vi "conector2.vi"(0 "salida":string[](array[string]), 1 "Salida ent":string, 2 "corriente entrada":dbl, 3 "polarizador":dbl[](array[numeric]), 4 "Polarizadorent":dbl, 5 "voltaje":dbl[](array[numeric]), 7 "VoltajeEnt":dbl, 8 "corrientes":dbl[](array[numeric]), 10 "Enum":T1(ring), 11 "Indice":i32) -> (12 "corrientes salida":dbl[](array[numeric]), 13 "VoltajeEnt 2":dbl, 14 "salida 2":string[](array[string]), 15 "Salida ent 2":string, 16 "corriente salida":dbl, 17 "polarizador 2":dbl[](array[numeric]), 18 "Polarizador":dbl, 19 "voltaje 2":dbl[](array[numeric]))   [LabVIEW 2016]
doc: "Este subVI selecciona al arreglo del cual se obtienen los valores que se enviarán a los dispositivos. \nLas entradas son tres arreglos y tres valores y de igual forma son las salidas."
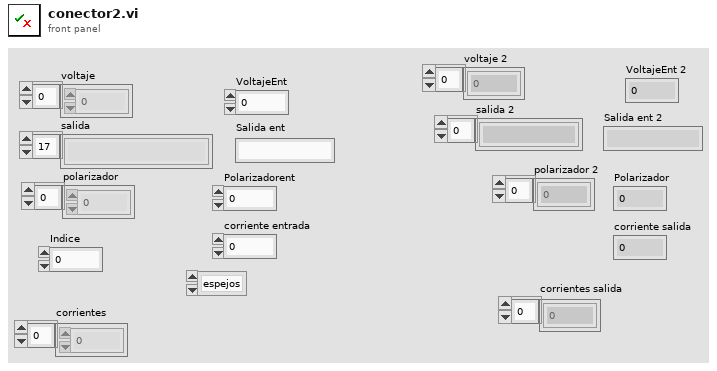
[diagram p1: front panel]
types:
  T1 = enum16{"espejos", "polarizador", "voltaje", "potenciometro ", "CCD", "lockin", "laser", "ninguno"}
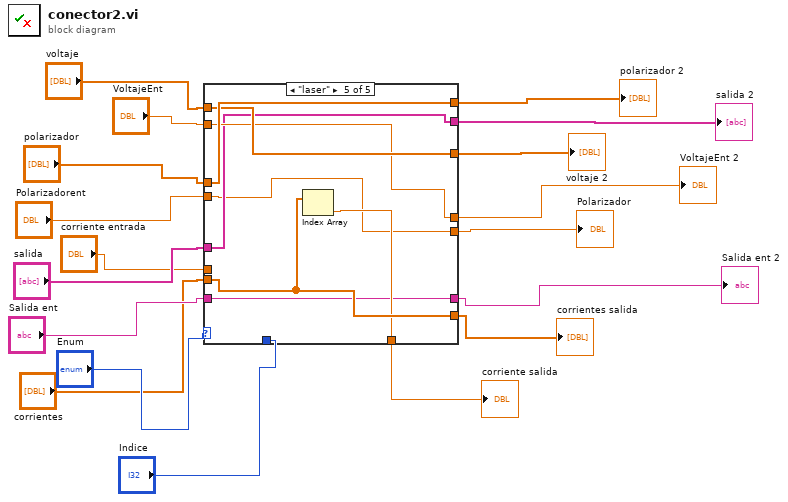
[diagram p0: block diagram]
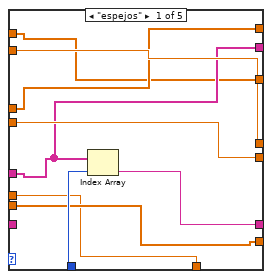
[diagram p2: hidden frame]
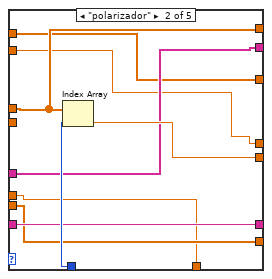
[diagram p3: hidden frame]
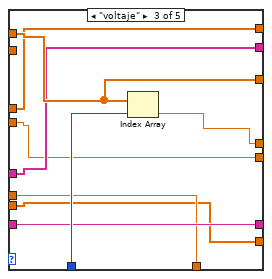
[diagram p4: hidden frame]
diagram:
  n1 = case shown="\"laser\"" "Enum" {
    tunnel: "polarizador" -> [w26 w34 w39 w53 w59]
    tunnel: "Indice" -> [w21 w36 w45 _ _]
    tunnel: [w25 w35 w40 w49 w55] -> w16
    tunnel: [w26 w34 w39 w53 w59] -> w15
    tunnel: "Polarizadorent" -> [w25 _ w40 w49 w55]
    tunnel: "salida" -> [w23 w33 w42 w52 w56]
    tunnel: "Salida ent" -> [_ w32 w41 w48 w54]
    tunnel: "VoltajeEnt" -> [w27 w31 _ w50 w57]
    tunnel: [w27 w31 w44 w50 w57] -> w10
    tunnel: [w24 w32 w41 w48 w54] -> w9
    tunnel: [w23 w33 w42 w52 w56] -> w8
    tunnel: "voltaje" -> [w22 w30 w43 w51 w58]
    tunnel: [w22 w30 w43 w51 w58] -> w6
    tunnel: "corrientes" -> [w20 w29 w37 w47 w61]
    tunnel: [w20 w29 w37 w47 w61] -> w3
    tunnel: [w19 w28 w38 w46 w60] -> w2
    tunnel: "corriente entrada" -> [w19 w28 w38 w46 _]
    frame "espejos" {
      n2 = Index Array(array=w23, index=w21) -> (element=w24:string)
    }
    frame "polarizador" {
      n3 = Index Array(array=w34, index=w36) -> (element=w35:dbl)
    }
    frame "voltaje" {
      n4 = Index Array(array=w43, index=w45) -> (element=w44:dbl)
    }
    frame "potenciometro ", Default {
    }
    frame "laser" {
      n5 = Index Array(array=w61) -> (element=w60:dbl)  [unwired: 1 in]
    }
  }
  "Polarizador" <- w16
  "polarizador 2" <- w15
  "VoltajeEnt 2" <- w10
  "Salida ent 2" <- w9
  "salida 2" <- w8
  "voltaje 2" <- w6
  "corriente salida" <- w2
  "corrientes salida" <- w3
